vi "Custom_Append VI Block Diagram to Report (path).vi"(0 "report in":refnum<class "NI_report.lvclass">, 1 "hidden frames":bool, 2 "image format (jpeg)":enum32{"PNG", "JPEG", "GIF"}(ring)=enum."JPEG", 5 "VI":path, 9 "alignment (default)":T2, 11 "error in (no error)":errorcluster, 12 "ordered (repeat from higher level if nested)":bool, 13 "MS Office parameters":T1) -> (4 "report out":refnum<class "NI_report.lvclass">, 6 "VI path out":path, 8 "start out (Word)":i32, 10 "end out (Word)":i32, 15 "error out":errorcluster)   [LabVIEW 2019]
doc: "Creates an image of the block diagram of the VI you specify in <B>VI</B> and appends the image to a report. Wire data to the <B>VI</B> input to determine the polymorphic instance to use or manually select the instance."
uses:
  <vilib>/Utility/NIReport.llb/NI_ReportGenerationCore.lvlib
  <vilib>/Utility/NIReport.llb/HTML Report Image Alignment.ctl
  <vilib>/Utility/NIReport.llb/NI_report.lvclass
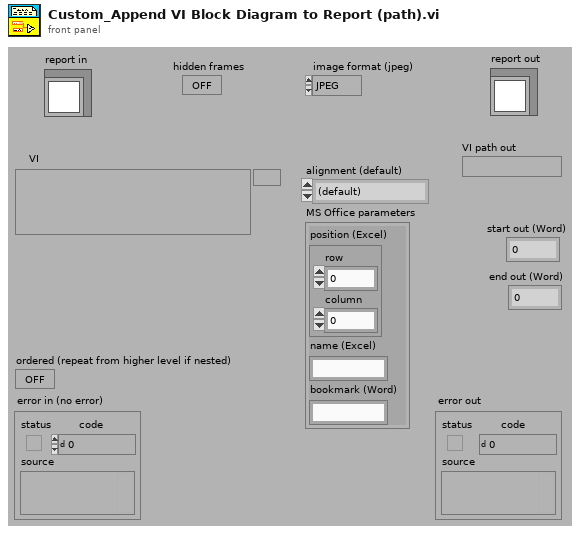
[diagram p1: front panel]
types:
  T1 = cluster{"position (Excel)":cluster{"row":i32, "column":i32}, "name (Excel)":string, "bookmark (Word)":string}
  T2 = typedef "NI_ReportGenerationCore.lvlib/HTML Report Image Alignment.ctl" = enum16{"(default)", "LEFT", "RIGHT", "TOP", "TEXTTOP", "MIDDLE", "ABSMIDDLE", "BASELINE", "BOTTOM", "ABSBOTTOM"}
  T3 = enum32{"invalid app kind", "Development System", "Run Time System", "Student Edition", "Embedded LabVIEW", "Evaluation", "Custom"}
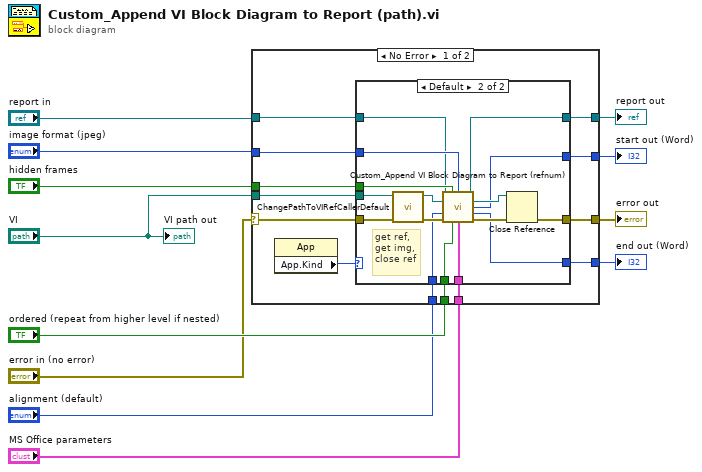
[diagram p0: block diagram]
diagram:
  n1 = case shown="No Error" "error in (no error)" {
    selector: "error in (no error)" -> [w21 w45]
    tunnel: [w18 w45] -> w5
    tunnel: [w15 w44] -> w6
    tunnel: "report in" -> [w14 w44]
    tunnel: "VI" -> [w22 _]
    tunnel: "image format (jpeg)" -> [w25 _]
    tunnel: "hidden frames" -> [w24 _]
    tunnel: "ordered (repeat from higher level if nested)" -> [w23 _]
    tunnel: "alignment (default)" -> [w20 _]
    tunnel: "MS Office parameters" -> [w19 _]
    tunnel: [w17 _] -> w2
    tunnel: [w16 _] -> w1
    frame No Error {
      n2 = property class="App"() -> ("App.Kind"=w13:T3)  [unwired: 2 in, 2 out]
      n3 = case shown="Default" w13 {
        tunnel: w25 -> [_ w43]
        tunnel: w24 -> [_ w42]
        tunnel: w23 -> [_ w41]
        tunnel: w22 -> [_ w40]
        tunnel: w21 -> [w27 w39]
        tunnel: w20 -> [_ w37]
        tunnel: w19 -> [_ w36]
        tunnel: [w27 w33] -> w18
        tunnel: [_ w32] -> w17
        tunnel: [_ w31] -> w16
        tunnel: [w26 w29] -> w15
        tunnel: w14 -> [w26 w28]
        frame "Run Time System" {
          # "Do not try to append\ndiagram if running\nin an executable"
        }
        frame Default {
          # "get ref,\nget img,\nclose ref"
          n4 = call <vilib>:"ChangePathToVIRefCallerDefault.vi"("error in (no error)"=w39, "VI path"=w40) -> ("error out"=w38:errorcluster, "VI reference"=w30:refnum<vi>)  [unwired: 4 in]
          n5 = call "Custom_Append VI Block Diagram to Report (refnum).vi"("report in"=w28, "hidden frames"=w42, "image format (jpeg)"=w43, "VI"=w30, "alignment (default)"=w37, "error in (no error)"=w38, "ordered (repeat from higher level if nested)"=w41, "MS Office parameters"=w36) -> ("report out"=w29:refnum<class "NI_report.lvclass">, "VI out"=w35:refnum<vi>, "start out (Word)"=w32:i32, "end out (Word)"=w31:i32, "error out"=w34:errorcluster)  [unwired: 3 in]
          n6 = Close Reference(reference=w35, error in (no error)=w34) -> (error out=w33:errorcluster)
        }
      }
    }
    frame Error {
    }
  }
  "error out" <- w5
  "report out" <- w6
  "start out (Word)" <- w2
  "end out (Word)" <- w1
  "VI path out" <- "VI"
